vi "Create.vi"(8 "error in (no error)":errorcluster, 9 "debug mode (F)":bool, 11 "Device Item Ref":T1=18446744073709551615 format="%.0x") -> (0 "error out":errorcluster, 3 "VeriStand Framework":refnum<class "VeriStand Data Sharing Framework.lvclass">)   [LabVIEW 2017, in "Data Sharing Framework Engine.lvlib" / "VeriStand Data Sharing Framework.lvclass"]
uses:
  VeriStand Data Sharing Framework.lvclass
  <vilib>/NI Veristand/Custom Device API/Custom Device Item Ref.ctl
  DSF Core.lvlibp/Engine/Classes/Framework/Framework Options.ctl
  DSF Core.lvlibp/Engine/Typedefs/FIFO Flags.ctl
  DSF Core.lvlibp/Engine/Classes/Thread/Thread Options.ctl
  DSF Core.lvlibp/Engine/Typedefs/Plugin Flags.ctl
  VeriStand Data Sharing Framework.lvclass/VeriStand Data Sharing Framework.ctl
  DSF Core.lvlibp
  DSF Core.lvlibp/Engine/Classes/Thread/Thread.lvclass
  DSF Core.lvlibp/Engine/Classes/Framework/Framework.lvclass
  DSF Core.lvlibp/DSF Configuration API/Configuration Session.lvclass
  <vilib>/NI Veristand/Custom Device API/Custom Device API.lvlib
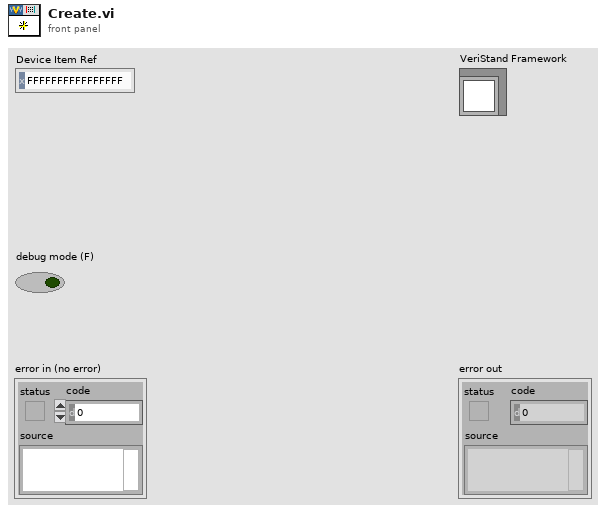
[diagram p1: front panel]
types:
  T1 = typedef "Custom Device API.lvlib/Custom Device Item Ref.ctl" = u64
  T2 = typedef "DSF Core.lvlibp/Framework.lvclass/Framework Options.ctl" = cluster{"FIFO Options":T3, "Thread Options":T4, "Plugin Options":T5}
  T3 = typedef "DSF Core.lvlibp/FIFO Flags.ctl" = cluster{"Infinite Timeouts":bool}
  T4 = typedef "DSF Core.lvlibp/Thread.lvclass/Thread Options.ctl" = cluster{"Show FP On Call":bool, "Close FP After Call":bool, "Allow Debugging":bool, "Show Menu Bar":bool, "Reposition Windows":bool}
  T5 = typedef "DSF Core.lvlibp/Plugin Flags.ctl" = cluster{"Default Components":bool}
  T6 = typedef "DSF Core.lvlibp/DSF Engine Framework Configuration.ctl" = cluster{"components directory":path, "Plugins":T7[]}
  T7 = typedef "DSF Core.lvlibp/DSF Engine Plugin Configuration.ctl" = cluster{"name":string, "components":string[], "cycle timing":T8, "threads":T9[], "Transfer Groups":T11[], "settings":T10}
  T8 = typedef "DSF Core.lvlibp/DSF Timing Info.ctl" = cluster{"priority":u64, "decimation":u64, "offset":u64}
  T9 = typedef "DSF Core.lvlibp/DSF Engine Plugin Thread Configuration.ctl" = cluster{"buffer converter settings":T10, "transceiver settings":T10, "processor":i32}
  T10 = typedef "DSF Core.lvlibp/DSF Settings Info.ctl" = cluster{"key":string, "value":string}[]
  T11 = typedef "DSF Core.lvlibp/DSF Engine Transfer Group Configuration.ctl" = cluster{"name":string, "direction":T12, "cycle timing":T8, "thread":i32, "settings":T10, "Transfers":T13[]}
  T12 = typedef "DSF Core.lvlibp/DSF Direction.ctl" = enum8{"Tx", "Rx"}
  T13 = typedef "DSF Core.lvlibp/DSF Engine Transfer Configuration.ctl" = cluster{"name":string, "byte order":T14, "channels":T15[], "settings":T10}
  T14 = typedef "DSF Core.lvlibp/DSF Byte Order.ctl" = enum8{"big-endian", "little-endian"}
  T15 = typedef "DSF Core.lvlibp/DSF Engine Channel Configuration.ctl" = cluster{"src buffer offset":u64, "name":string, "data type":T16, "count":u64, "dst buffer offset":u64}
  T16 = typedef "DSF Core.lvlibp/DSF Data Type.ctl" = enum8{"Bool", "SGL", "DBL", "I8", "I16", "I32", "I64", "U8", "U16", "U32", "U64"}
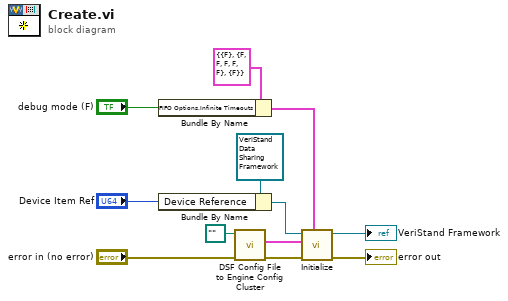
[diagram p0: block diagram]
diagram:
  n1 = Bundle By Name(cluster=T2 {"FIFO Options"={"Infinite Timeouts"=FALSE}, "Thread Options"={"Show FP On Call"=FALSE, "Close FP After Call"=FALSE, "Allow Debugging"=FALSE, "Show Menu Bar"=FALSE, "Reposition Windows"=FALSE}, "Plugin Options"={"Default Components"=FALSE}} ("options"), "FIFO Options.Infinite Timeouts"="debug mode (F)") -> (w9:T2)
  n2 = Bundle By Name(cluster=refnum<class "VeriStand Data Sharing Framework.lvclass"> refnum ("VeriStand DSF.Framework.lvclass"), "Device Reference"="Device Item Ref") -> (w3:refnum<class "VeriStand Data Sharing Framework.lvclass">)
  n3 = call "DSF Config File to Engine Config Cluster.vi"("error in (no error)"="error in (no error)", "dsf configuration file path"=path "") -> ("error out"=w7:errorcluster, "framework configuration out"=w2:T6)  [unwired: 7 in, 1 out]
  n4 = call-dynamic "Initialize.vi"("options"=w9, "error in (no error)"=w7, "framework configuration"=w2, "VeriStand Data Sharing Framework in"=w3) -> ("error out"=→"error out":errorcluster, "VeriStand Data Sharing Framework out"=→"VeriStand Framework":refnum<class "VeriStand Data Sharing Framework.lvclass">)  [unwired: 6 in]
